vi "Thermometer.vi"(1 "Units (0: Celsius)":u16(ring) items=["Celsius", "Fahrenheit"]) -> (0 "Temperature":dbl(slide) scale=0.0..100.0)   [LabVIEW 2014]
doc: "This VI measures temperature using the temperature sensor on the DAQ BNC-2120 terminal block."
uses:
  Instance           1 19Saved   Thermometer .vi
  Instance           2 19Saved   Thermometer .vi
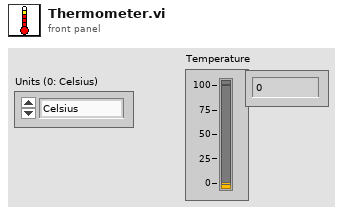
[diagram p1: front panel]
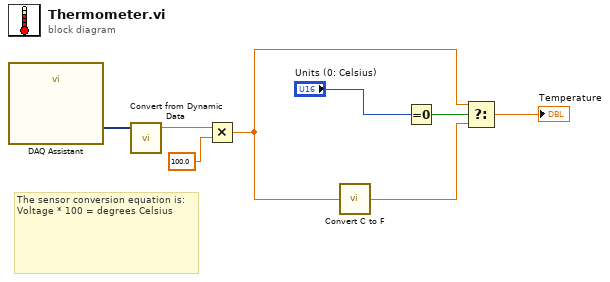
[diagram p0: block diagram]
diagram:
  # "The sensor conversion equation is: \nVoltage * 100 = degrees Celsius"
  n1 = call "DAQ Assistant"() -> ("data"=w7:dynamicdata)  [unwired: 17 in, 2 out]
  n2 = call "Convert from Dynamic Data"("Dynamic Data Type"=w7) -> ("Scalar"=w5:dbl)  [unwired: 3 in]
  n3 = Multiply(x=w5, y=100.0) -> (x*y=w6:dbl)
  n4 = call "Convert C to F.vi"("Degrees Celsius"=w6) -> ("Degrees Fahrenheit"=w8:dbl)
  n5 = Equal To 0?(x="Units (0: Celsius)") -> (x = 0?=w1:bool)
  n6 = Select(t=w6, s=w1, f=w8) -> (s? t:f=→"Temperature":dbl)
